vi "RemovenearestROI.vi"(4 "Cursor.Cursor Position":T1, 8 "ROI array in":u32[][](array[numeric])) -> (2 "ROI array out 2":u32[][](array[numeric]))   [LabVIEW 2011, in "OfflineTracker.lvlib"]
uses:
  <vilib>/Utility/miscctls.llb/LVPointDoubleTypeDef.ctl
  OfflineTracker.lvlib
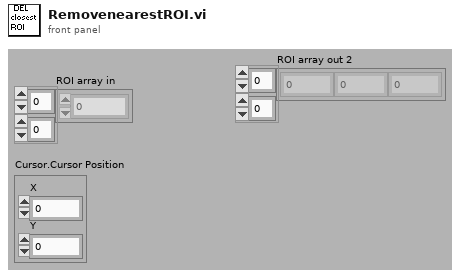
[diagram p1: front panel]
types:
  T1 = typedef "LVPointDoubleTypeDef.ctl" = cluster{"X":dbl, "Y":dbl}
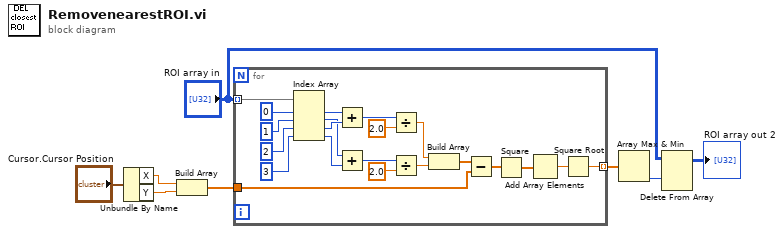
[diagram p0: block diagram]
diagram:
  n1 = Unbundle By Name("Cursor.Cursor Position") -> ("X"=w7:dbl, "Y"=w6:dbl)
  n2 = Build Array(w7, w6) -> (w5:dbl[])
  n3 = for {
    tunnel: "ROI array in" -> [w29] mode=indexing
    tunnel: w5 -> [w13]
    tunnel: [w9] -> w4 mode=indexing
    n4 = Index Array(array=w29, index #1=0 ("index"), index #2=1 ("index"), index #3=2 ("index"), index #4=3 ("index")) -> (element #1=w22:u32, element #2=w20:u32, element #3=w21:u32, element #4=w19:u32)
    n5 = Add(x=w22, y=w21) -> (x+y=w18:u32)
    n6 = Add(x=w20, y=w19) -> (x+y=w17:u32)
    n7 = Divide(x=w18, y=2.0) -> (x/y=w16:dbl)
    n8 = Divide(x=w17, y=2.0) -> (x/y=w15:dbl)
    n9 = Build Array(w16, w15) -> (w14:dbl[])
    n10 = Subtract(x=w14, y=w13) -> (x-y=w12:dbl[])
    n11 = Square(x=w12) -> (x^2=w11:dbl[])
    n12 = Add Array Elements(numeric array=w11) -> (sum=w10:dbl)
    n13 = Square Root(x=w10) -> (sqrt(x)=w9:dbl)
  }
  n14 = Array Max & Min(array=w4) -> (min index (indices)=w2:i32)  [unwired: 3 out]
  n15 = Delete From Array(array="ROI array in", index (row)=w2) -> (array with subset deleted=→"ROI array out 2":u32[][])  [unwired: 2 in, 1 out]
